vi "WPI_CompressorControlLoop.vi"(8 "error in (no error)":errorcluster, 10 "CompressorDevRef 2":T1={"DevStatus"={"status"=FALSE, "code"=0, "source"=""}, "DigitalInputDevRef"={"DevStatus"={"status"=FALSE, "code"=0, "source"=""}, "DIO Channel"=enum."Invalid", "Controller"=enum."Controller 1"}, "RelayDevRef"={"DevStatus"={"status"=FALSE, "code"=0, "source"=""}, "Relay Channel"=enum."Invalid", "Controller"=enum."Controller 1", "Relay Direction"=enum."Both directions"}}, 11 "CompressorDevRef":T1={"DevStatus"={"status"=FALSE, "code"=0, "source"=""}, "DigitalInputDevRef"={"DevStatus"={"status"=FALSE, "code"=0, "source"=""}, "DIO Channel"=enum."Invalid", "Controller"=enum."Controller 1"}, "RelayDevRef"={"DevStatus"={"status"=FALSE, "code"=0, "source"=""}, "Relay Channel"=enum."Invalid", "Controller"=enum."Controller 1", "Relay Direction"=enum."Both directions"}}) -> ()   [LabVIEW 2014, in "hhVI.lvlib"]
doc: "Monitors the pressure switch and updates the relay of up to two compressors. Use the Start, Stop, and GetEnableState VIs to update the compressor state. Use this VI in parallel with the rest of the robot code. Do not place this VI in another loop or in the Teleop code.\n\nThis software is licensed. Open the labview\\readme\\WPI Robotics Library Open Source License.txt file for more information."
uses:
  hhVI.lvlib
  <vilib>/Rock Robotics/WPI/Relay/WPI_RelayValue.ctl
  <vilib>/Rock Robotics/SystemInterfaces/DIO/FPGA_DIOChannel.ctl
  <vilib>/Rock Robotics/SystemInterfaces/Typedef/FPGA_TypedefDigitalModule.ctl
  <vilib>/Rock Robotics/WPI/DigitalInput/WPI_DigitalInputDevRef.ctl
  <vilib>/Rock Robotics/SystemInterfaces/DIO/FPGA_DIORelayChannel.ctl
  <vilib>/Rock Robotics/WPI/Relay/WPI_RelayDirection.ctl
  <vilib>/Rock Robotics/WPI/Relay/WPI_RelayDevRef.ctl
  <vilib>/Rock Robotics/WPI/Compressor/WPI_CompressorDevRef.ctl
panel:
  # "This VI loops and doesn't return.\nPlacing it into another loop will\nprevent that loop from iterating.\n\nPeriodic tasks is a good location for it."
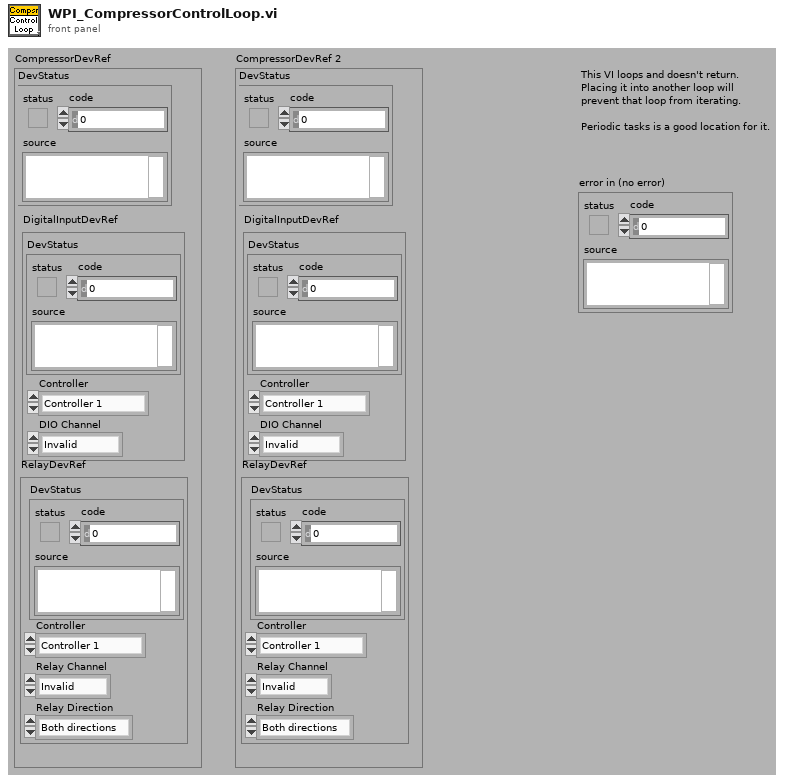
[diagram p1: front panel]
types:
  T1 = typedef "WPI_CompressorDevRef.ctl" = cluster{"DevStatus":errorcluster, "DigitalInputDevRef":T2, "RelayDevRef":T5}
  T2 = typedef "WPI_DigitalInputDevRef.ctl" = cluster{"DevStatus":errorcluster, "DIO Channel":T3, "Controller":T4}
  T3 = typedef "FPGA_DIOChannel.ctl" = enum8{"DIO 0", "DIO 1", "DIO 2", "DIO 3", "DIO 4", "DIO 5", "DIO 6", "DIO 7", "DIO 8", "DIO 9", "DIO MXP 0", "DIO MXP 1", "DIO MXP 2", "DIO MXP 3", "DIO MXP 4", "DIO MXP 5", "DIO MXP 6", "DIO MXP 7", "DIO MXP 8", "DIO MXP 9", "DIO MXP 10", "DIO MXP 11", "DIO MXP 12", "DIO MXP 13", "DIO MXP 14", "DIO MXP 15", "Invalid"}
  T4 = typedef "FPGA_TypedefDigitalModule.ctl" = enum16{"Controller 1"}
  T5 = typedef "WPI_RelayDevRef.ctl" = cluster{"DevStatus":errorcluster, "Relay Channel":T6, "Controller":T4, "Relay Direction":T7}
  T6 = typedef "FPGA_DIORelayChannel.ctl" = enum8{"Relay 0", "Relay 1", "Relay 2", "Relay 3", "Invalid"}
  T7 = typedef "WPI_RelayDirection.ctl" = enum16{"Both directions", "Forward only", "Reverse only"}
  T8 = typedef "WPI_RelayValue.ctl" = enum16{"Off", "On", "Forward", "Reverse"}
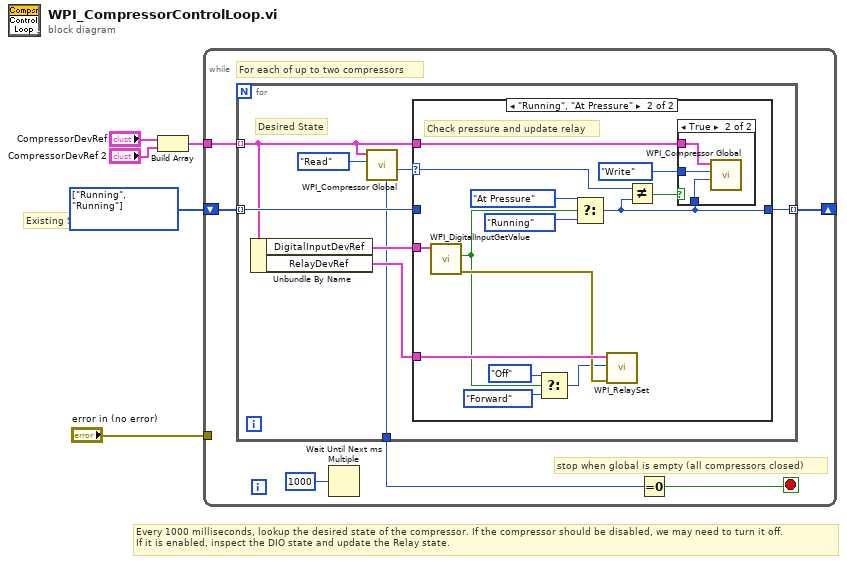
[diagram p0: block diagram]
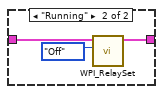
[diagram p3: hidden frame]
diagram:
  w1 = enum16{"Disabled", "Running", "At Pressure"}[] [enum."Running", enum."Running"] items=["Disabled", "Running", "At Pressure"]
  # "Every 1000 milliseconds, lookup the desired state of the compressor. If the compressor should be disabled, we may need to turn it off.\nIf it is enabled, inspect the DIO state and update the Relay state."
  # "Existing State"
  n1 = Build Array("CompressorDevRef", "CompressorDevRef 2") -> (w4:T1[])
  n2 = while {
    shift-right: [w9] -> _
    shift-left: w1 -> [w10]
    tunnel: "error in (no error)" -> [_]
    tunnel: w4 -> [w8]
    stop <- w6 stop-if-true
    # "stop when global is empty (all compressors closed)"
    # "For each of up to two compressors"
    n3 = for {
      tunnel: w10 -> [w19] mode=indexing
      tunnel: [w18] -> w9 mode=indexing
      tunnel: w8 -> [w13] mode=indexing
      tunnel: [w12] -> w7
      # "Desired State"
      n4 = Unbundle By Name(w13) -> ("DigitalInputDevRef"=w15:T2, "RelayDevRef"=w14:T5)
      n5 = call <vilib>:"WPI_Compressor Global.vi"("Operation"=enum16{"Read", "Write", "Add", "Remove"}."Read", "CompressorDevRef"=w13) -> ("Compressor State Out"=w16:enum16{"Disabled", "Running", "At Pressure"}, "Compressor Count"=w12:u8)  [unwired: 8 in]
      n6 = case shown="\"Running\", \"At Pressure\"" w16 {
        selector: w16 -> [w20 w27]
        tunnel: w15 -> [_ w40]
        tunnel: w14 -> [w22 w39]
        tunnel: w19 -> [w21 _]
        tunnel: [w20 w28] -> w18
        tunnel: w13 -> [_ w30]
        frame "Disabled", Default {
          n7 = case shown="Default" w21 {
            tunnel: w22 -> [w23 w25]
            tunnel: [w23 w24] -> _
            frame Default {
            }
            frame "Running" {
              n8 = call <vilib>:"WPI_RelaySet.vi"("RelayValue"=WPI_RelayValue."Off", "RelayDevRef"=w25) -> ("RelayDevRef"=w24:T5)  [unwired: 1 in, 8 out]
            }
          }
        }
        frame "Running", "At Pressure" {
          # "Check pressure and update relay"
          n9 = call <vilib>:"WPI_DigitalInputGetValue.vi"("DigitalInputDevRef"=w40) -> ("error out"=w38:errorcluster, "Value"=w34:bool)  [unwired: 1 in, 8 out]
          n10 = Select(t=WPI_RelayValue."Off" ("RelayValue"), s=w34, f=WPI_RelayValue."Forward" ("RelayValue")) -> (s? t:f=w35:T8)
          n11 = Select(t=enum16{"Disabled", "Running", "At Pressure"}."At Pressure" ("Compressor State"), s=w34, f=enum16{"Disabled", "Running", "At Pressure"}."Running" ("Compressor State")) -> (s? t:f=w28:enum16{"Disabled", "Running", "At Pressure"})
          n12 = call <vilib>:"WPI_RelaySet.vi"("error in (no error)"=w38, "RelayValue"=w35, "RelayDevRef"=w39) -> ()  [unwired: 9 out]
          n13 = Not Equal?(x=w27, y=w28) -> (x != y?=w29:bool)
          n14 = case shown="True" w29 {
            tunnel: w28 -> [_ w43]
            tunnel: enum16{"Read", "Write", "Add", "Remove"}."Write" ("Operation") -> [_ w42]
            tunnel: w30 -> [_ w41]
            frame False {
            }
            frame True {
              n15 = call <vilib>:"WPI_Compressor Global.vi"("Compressor State In"=w43, "Operation"=w42, "CompressorDevRef"=w41) -> ()  [unwired: 7 in, 2 out]
            }
          }
        }
      }
    }
    n16 = Wait Until Next ms Multiple(millisecond multiple=u32 1000 ("timeout in ms (0)")) -> ()  [unwired: 1 out]
    n17 = Equal To 0?(x=w7) -> (x = 0?=w6:bool)
  }
